vi "类型2自动测试结果.vi"(8 "合格?":bool, 11 "第几组":i32) -> ()   [LabVIEW 2010]
uses:
  全局量/自动测试结果.vi
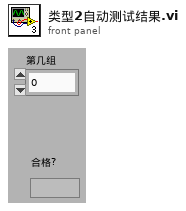
[diagram p1: front panel]
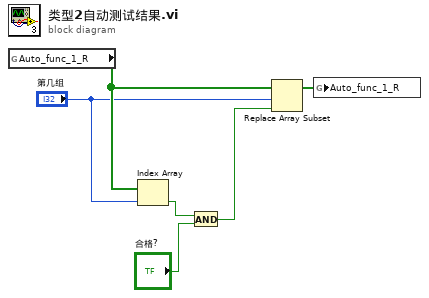
[diagram p0: block diagram]
diagram:
  n1 = global read "自动测试结果.vi" "Auto_func_1_R"() -> (w4:bool[])
  n2 = Index Array(array=w4, index="第几组") -> (element=w6:bool)
  n3 = And(x=w6, y="合格?") -> (x .and. y?=w1:bool)
  n4 = Replace Array Subset(array=w4, new element=w1, index="第几组") -> (w3:bool[])
  n5 = global write "自动测试结果.vi" "Auto_func_1_R"(w3) -> ()
